vi "_Run Engine Server.vi"() -> ()   [LabVIEW 2015]
uses:
  Type/_Run State.ctl
  Type/_Log Command.ctl
  Type/_File Command.ctl
  Type/_RT Command.ctl
  Configuration/AcquisitionState.ctl
  _Server Global.vi
  Configuration/_Global Configuration.vi
panel:
  out "appended array":i32[](array[numeric])
  out "size(s)":i32
  out "first subarray":i32[](array[numeric])
  out "Remaining Scans":i32
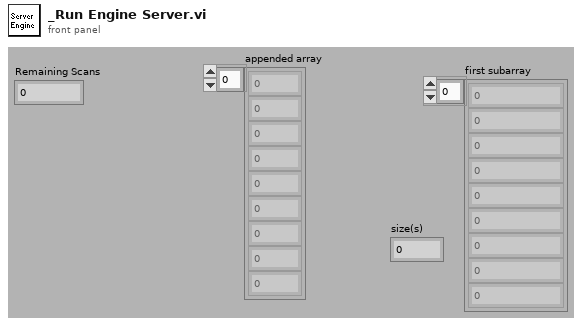
[diagram p1: front panel]
types:
  T1 = typedef "_Run State.ctl" = enum16{"Init", "Update", "Start", "End", "Error"}
  T2 = typedef "_Log Command.ctl" = enum16{"No Command", "Open", "Read", "Write", "Close", "Check Size"}
  T3 = typedef "_File Command.ctl" = enum16{"No Command", "Open", "Open Read", "Write", "Get Spectrum", "Close"}
  T4 = typedef "_RT Command.ctl" = enum16{"xml Start Run", "xml Start Actual Run", "xml Stop Run", "xml Runtime Update", "xml Get Status", "xml Get Table", "xml Set Table", "xml Get Configuration", "xml System Status", "xml Set LC Input Logic", "xml Get Data", "xml Get Info", "Start", "StartActualRun", "Stop", "Runtime Update", "Get Data", "Get Info", "Get Status", "Get Param", "Get Config", "Get Table", "Read ADC", "Set Oscillator", "Update Config", "Update Table", "Set All Pol", "Set Pol and DC", "Set Max Mass", "Toggle RP", "Toggle EL", "Set PIC", "Initialize Turbo", "Send Turbo Comm", "Close Turbo", "P1", "P2", "P3", "Send Serial", "Set LC Out", "Get LC In", "Read VAC", "Test Table", "Toggle Power", "Get Startup", "Set Startup", "Get ADC Table", "Set ADC Table", "Get Brief Status", "Get Detail Status", "Auxiliary Update", "Set CC Logics", "Set CC Input Logics", "Ignore Error", "invalid"}
  T5 = typedef "AcquisitionState.ctl" = enum16{"Ready", "Busy", "Waiting"}
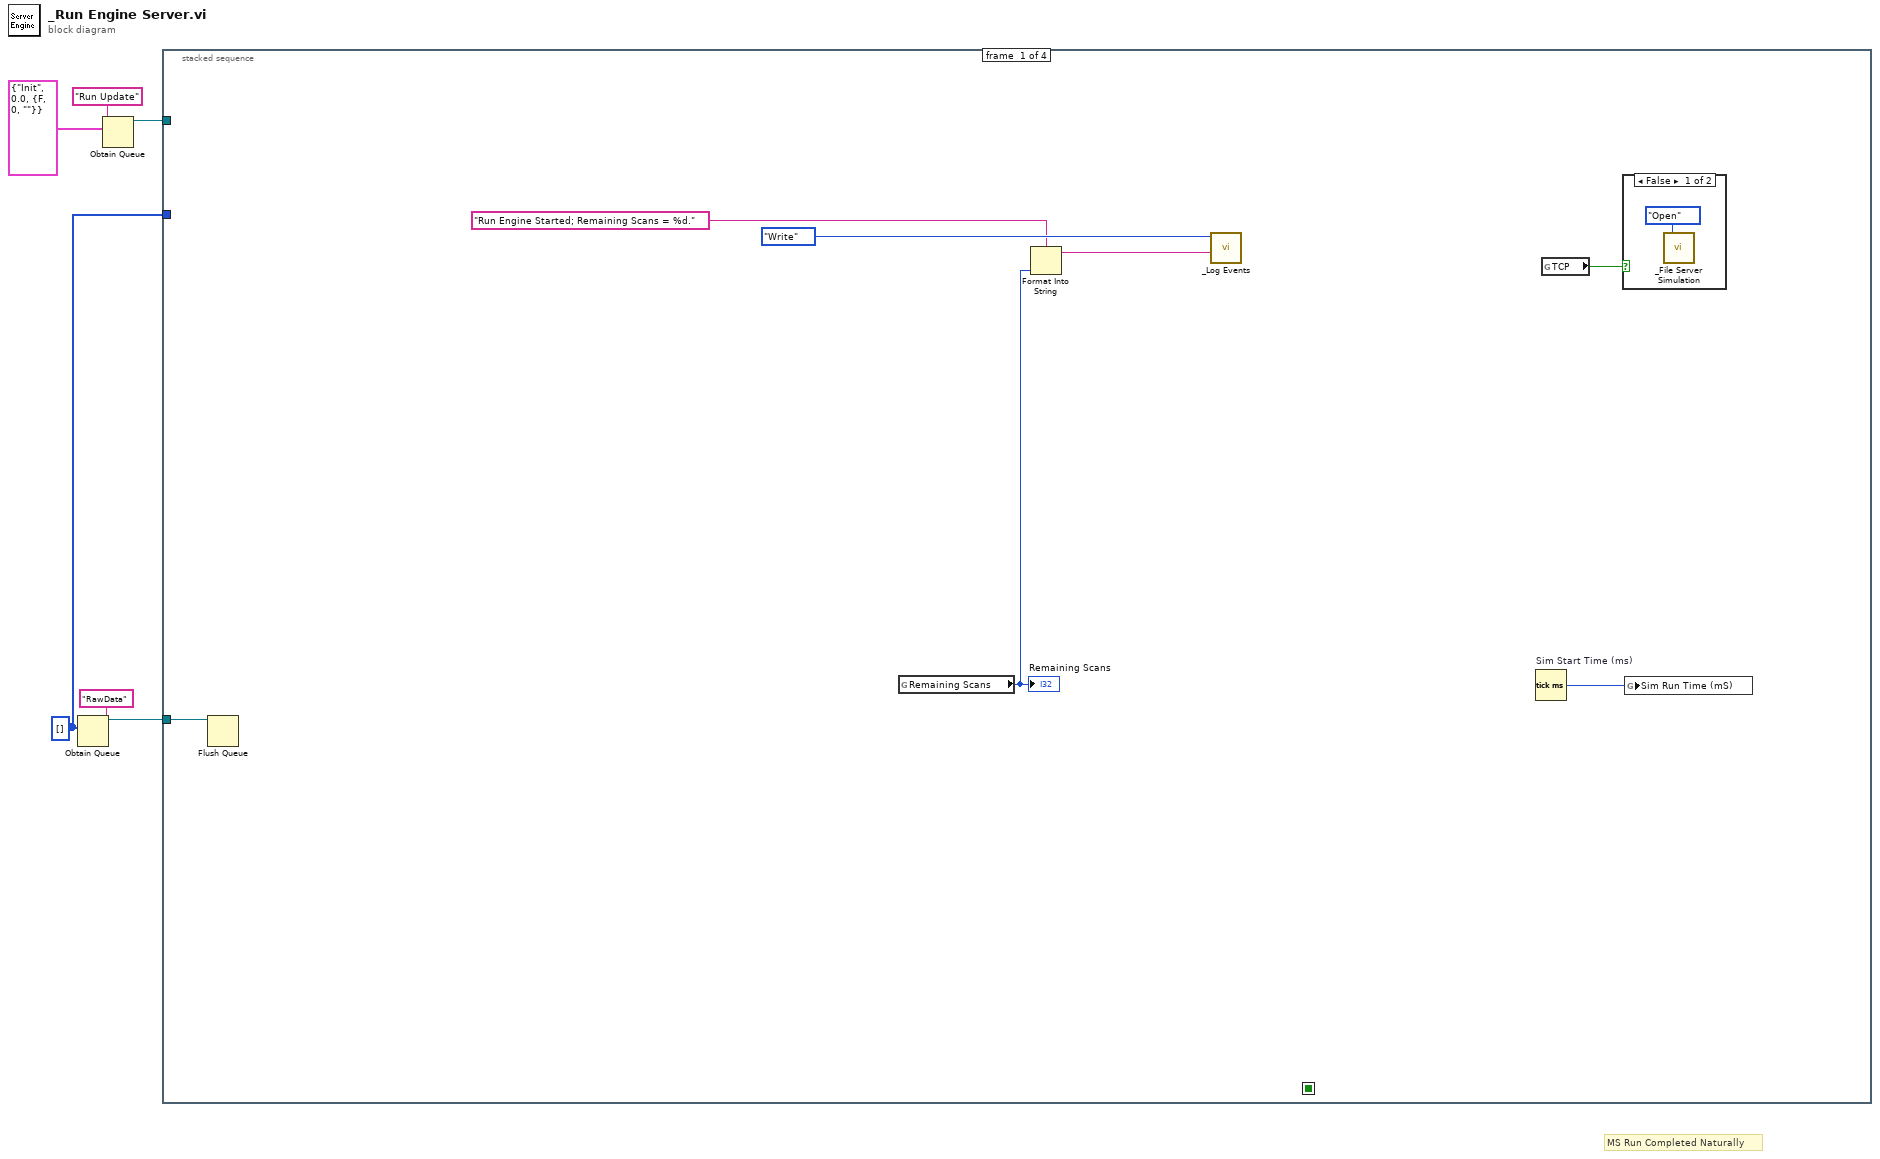
[diagram p0: block diagram]
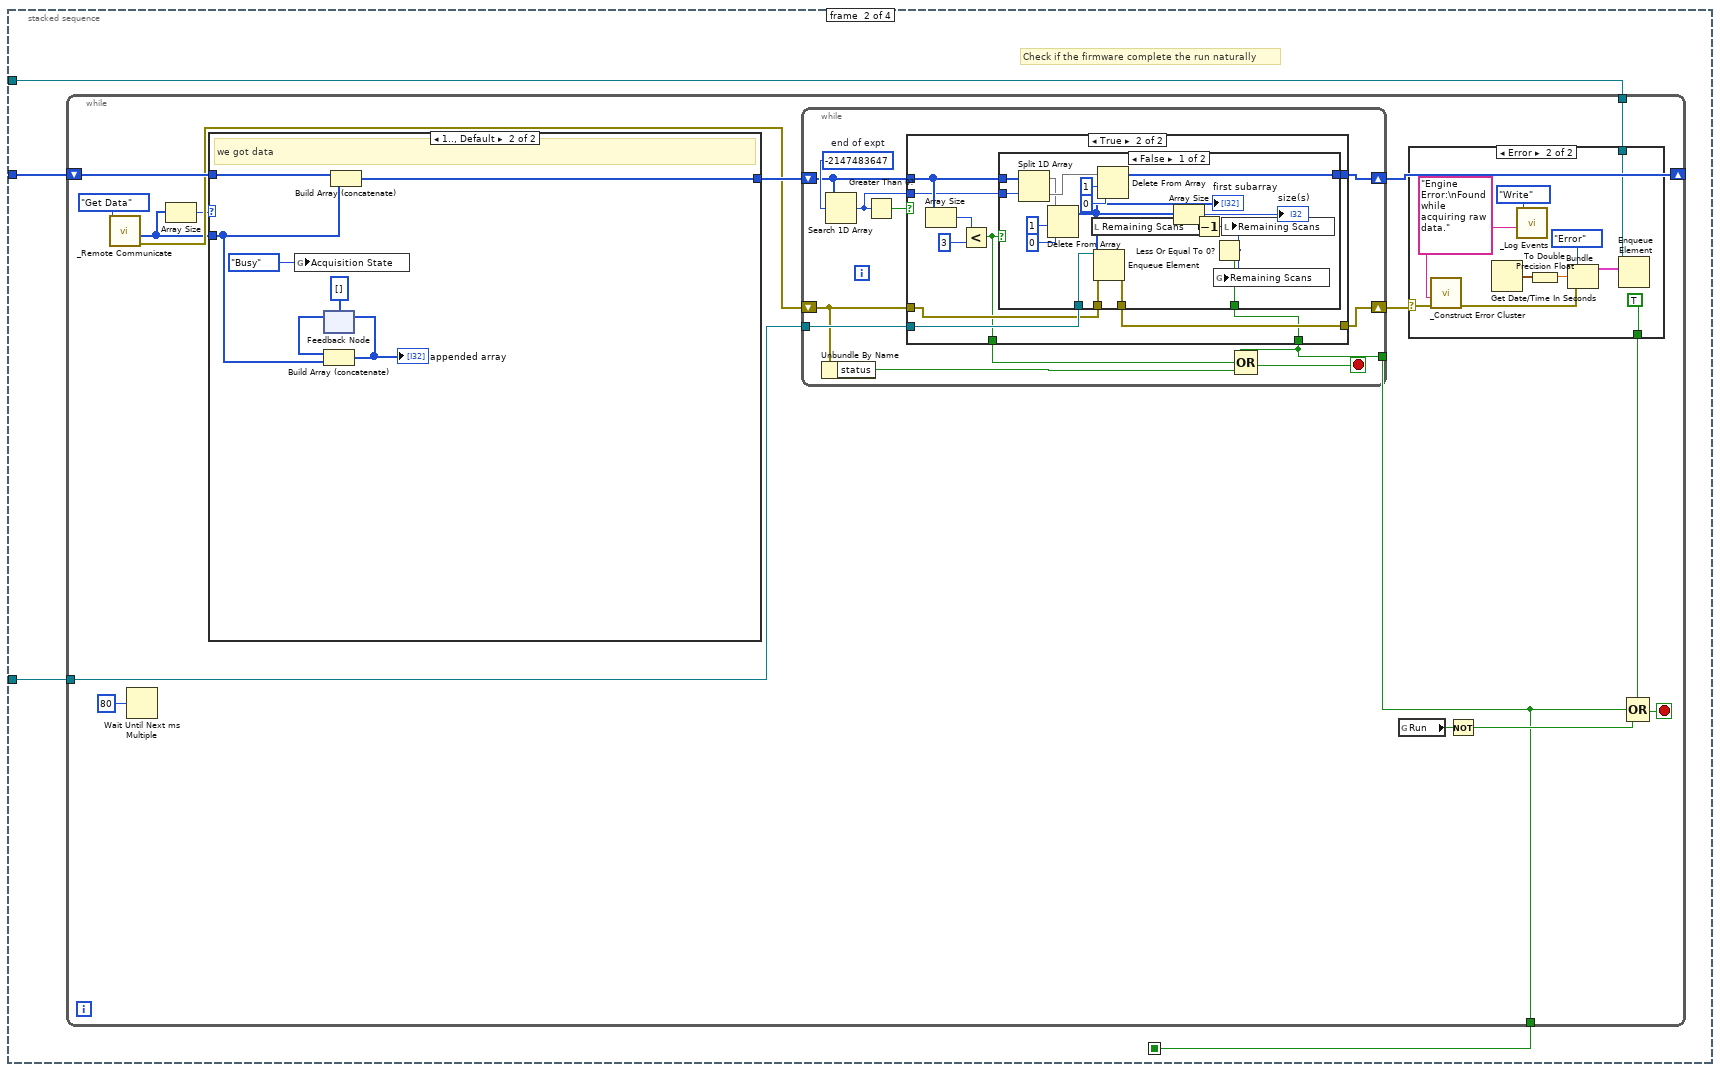
[diagram p3: hidden frame]
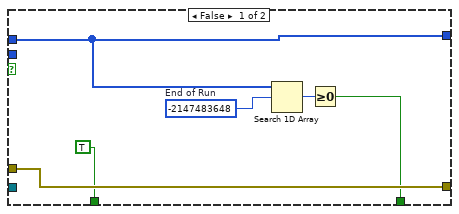
[diagram p5: hidden frame]
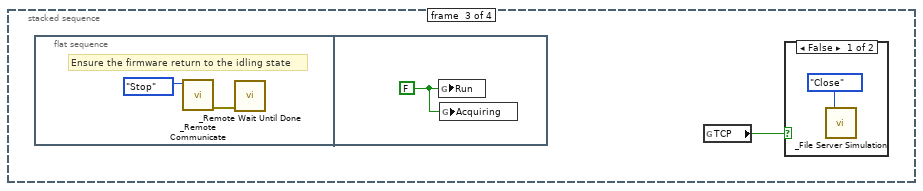
[diagram p8: hidden frame]
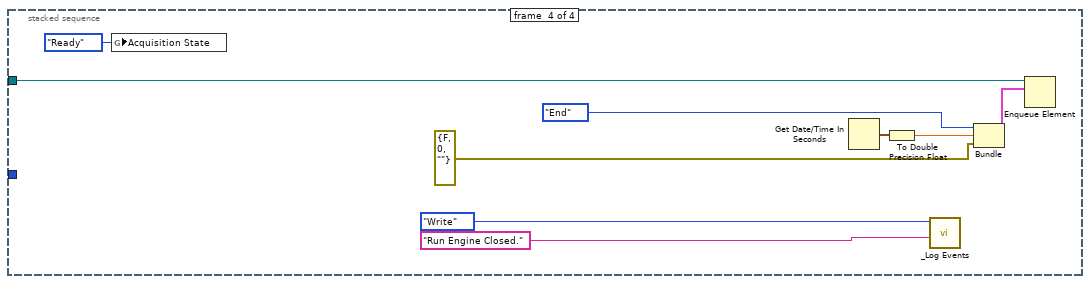
[diagram p10: hidden frame]
diagram:
  w4 = i32[] []
  # "MS Run Completed Naturally"
  n1 = Obtain Queue(name (unnamed)="RawData", element data type=w4) -> (queue out=w5:refnum<queue>)  [unwired: 3 in, 2 out]
  n2 = Obtain Queue(name (unnamed)="Run Update", element data type=cluster{T1, dbl, "error out":errorcluster} {enum."Init", 0.0, "error out"={"status"=FALSE, "code"=0, "source"=""}}) -> (queue out=w1:refnum<queue>)  [unwired: 3 in, 2 out]
  n3 = stacked-sequence {
    seq-local: [_ w15 _ _] -> [_ _ _ _]
    tunnel: w5 -> [w13 w18 _ _]
    tunnel: w4 -> [_ w17 _ _]
    tunnel: w1 -> [_ w16 _ w108]
    frame #0 {
      n4 = Flush Queue(queue=w13) -> ()  [unwired: 1 in, 3 out]
      n5 = global read "_Server Global.vi" "Remaining Scans"() -> (w11:i32)
      "Remaining Scans" <- w11
      n6 = Format Into String(format string="Run Engine Started; Remaining Scans = %d.", w11) -> (resulting string=w9:string)  [unwired: 2 in, 1 out]
      n7 = call "_Log Events.vi"("Event"=w9, "Log Command"=_Log_Command."Write") -> ()  [unwired: 6 in, 2 out]
      n8 = Tick Count (ms) "Sim Start Time (ms)"() -> (millisecond timer value=w7:u32)
      n9 = global read "_Global Configuration.vi" "TCP"() -> (w8:bool)
      n10 = case shown="False" w8 {
        frame False {
          n11 = call "_File Server Simulation.vi"("FileCommand"=_File_Command."Open") -> ()  [unwired: 1 in, 2 out]
        }
        frame True {
        }
      }
      n12 = global write "_Server Global.vi" "Sim Run Time (mS)"(w7) -> ()
    }
    frame #1 {
      # "Check if the firmware complete the run naturally"
      n13 = while {
        tunnel: w18 -> [w33]
        shift-right: [w27] -> _
        shift-left: w17 -> [w26]
        tunnel: w16 -> [w22]
        tunnel: [w21] -> w15
        stop <- w32 stop-if-true
        n14 = call "_Remote Communicate.vi"("Command"=_RT_Command."Get Data") -> ("error out"=w24:errorcluster, "Data Array"=w20:i32[])  [unwired: 5 in, 2 out]
        n15 = Wait Until Next ms Multiple(millisecond multiple=u32 80) -> ()  [unwired: 1 out]
        n16 = Array Size(array=w20) -> (size(s)=w19:i32)
        n17 = case shown="1.., Default" w19 {
          tunnel: w26 -> [w35 w42]
          tunnel: [w35 w41] -> w25
          tunnel: w20 -> [_ w36]
          frame 0 {
            # "nothing yet"
          }
          frame 1.., Default {
            # "we got data"
            n18 = global write "_Global Configuration.vi" "Acquisition State"(AcquisitionState."Busy" ("Acquisition State")) -> ()
            n19 = feedback #1(i32[] []) -> (w39:i32[])
            n20 = Build Array (concatenate)(w39, w36) -> (w38:i32[])
            "appended array" <- w38
            n21 = feedback-in #1(w38) -> ()
            n22 = Build Array (concatenate)(w42, w36) -> (w41:i32[])
          }
        }
        n23 = while {
          tunnel: w33 -> [w54]
          tunnel: [w46] -> w21
          shift-right: [w52] -> w27
          shift-left: w25 -> [w50]
          shift-right: [w53] -> w29
          shift-left: w24 -> [w48]
          stop <- w44 stop-if-true
          w51 = -2147483647  # end of expt
          n24 = Unbundle By Name(w48) -> ("status"=w45:bool)
          n25 = Search 1D Array(1D array=w50, element=w51) -> (index of element=w49:i32)  [unwired: 1 out]
          n26 = Greater Than 0?(x=w49) -> (x > 0?=w47:bool)
          n27 = case shown="True" w47 {
            tunnel: w48 -> [w60 w68]
            tunnel: w54 -> [_ w69]
            tunnel: [w60 w67] -> w53
            tunnel: w50 -> [w57 w63]
            tunnel: [w57 w70] -> w52
            tunnel: [w56 w66] -> w46
            tunnel: w49 -> [_ w62]
            tunnel: [TRUE w61] -> w43
            frame False {
              w58 = -2147483648  # End of Run
              n28 = Search 1D Array(1D array=w57, element=w58) -> (index of element=w59:i32)  [unwired: 1 out]
              n29 = Greater Or Equal To 0?(x=w59) -> (x >= 0?=w56:bool)
            }
            frame True {
              n30 = Array Size(array=w63) -> (size(s)=w65:i32)
              n31 = Less?(x=w65, y=3) -> (x < y?=w61:bool)
              n32 = case shown="False" w61 {
                tunnel: w63 -> [w87 w88]
                tunnel: w62 -> [w86 _]
                tunnel: [w79 w88] -> w70
                tunnel: w69 -> [w82 _]
                tunnel: w68 -> [w81 w89]
                tunnel: [w80 w89] -> w67
                tunnel: [w72 _] -> w66
                frame False {
                  n33 = Split 1D Array(array=w87, index=w86) -> (first subarray=w74:i32[], second subarray=w84:i32[])
                  n34 = Delete From Array(array=w74, length=1, index=0) -> (array with subset deleted=w73:i32[])  [unwired: 1 out]
                  "first subarray" <- w73
                  n35 = local read "Remaining Scans"() -> (w78:i32)
                  n36 = Enqueue Element(queue=w82, element=w73, error in (no error)=w81) -> (error out=w80:errorcluster)  [unwired: 3 out]
                  n37 = Delete From Array(array=w84, length=1, index=0) -> (array with subset deleted=w79:i32[])  [unwired: 1 out]
                  n38 = Array Size(array=w73) -> (size(s)=→"size(s)":i32)
                  n39 = Decrement(x=w78) -> (x-1=w71:i32)
                  n40 = Less Or Equal To 0?(x=w71) -> (x <= 0?=w72:bool)
                  n41 = global write "_Server Global.vi" "Remaining Scans"(w71) -> ()
                  n42 = local write "Remaining Scans"(w71) -> ()
                }
                frame True {
                }
              }
            }
          }
          n43 = Compound Arithmetic op=OR(w46, w43, w45) -> (w44:bool)
        }
        n44 = global read "_Global Configuration.vi" "Run"() -> (w31:bool)
        n45 = case shown="Error" w29 {
          selector: w29 -> [_ w99]
          tunnel: [_ TRUE] -> w28
          tunnel: w22 -> [_ w92]
          frame No Error {
          }
          frame Error {
            w90 = "Engine Error:\nFound while  acquiring raw data." ("format string")
            n46 = call "_Construct Error Cluster.vi"("error in"=w99, "reason"=w90) -> ("error out"=w95:errorcluster)  [unwired: 2 in, 3 out]
            n47 = Get Date/Time In Seconds() -> (seconds since 1Jan1904=w94:timestamp)
            n48 = call "_Log Events.vi"("Event"=w90, "Log Command"=_Log_Command."Write" ("File Command")) -> ()  [unwired: 6 in, 2 out]
            n49 = To Double Precision Float(number=w94) -> (double precision float=w93:dbl)
            n50 = Bundle(_Run_State."Error", w93, "error out"=w95) -> (w97:cluster{T1, dbl, "error out":errorcluster})  [unwired: 1 out]
            n51 = Enqueue Element(queue=w92, element=w97) -> ()  [unwired: 1 in, 4 out]
          }
        }
        n52 = Not(x=w31) -> (.not. x?=w30:bool)
        n53 = Compound Arithmetic op=OR(w28, w21, w30) -> (w32:bool)
      }
    }
    frame #2 {
      n54 = flat-sequence {
        frame #0 {
          # "Ensure the firmware return to the idling state"
          n55 = call "_Remote Communicate.vi"("Command"=_RT_Command."Stop") -> ("error out"=w103:errorcluster)  [unwired: 5 in, 3 out]
          n56 = call "_Remote Wait Until Done.vi"("error IO"=w103) -> ()  [unwired: 1 in, 2 out]
        }
        frame #1 {
          w104 = FALSE ("Update")
          n57 = global write "_Global Configuration.vi" "Run"(w104) -> ()
          n58 = global write "_Global Configuration.vi" "Acquiring"(w104) -> ()
        }
      }
      n59 = global read "_Global Configuration.vi" "TCP"() -> (w100:bool)
      n60 = case shown="False" w100 {
        frame False {
          n61 = call "_File Server Simulation.vi"("FileCommand"=_File_Command."Close") -> ()  [unwired: 1 in, 2 out]
        }
        frame True {
        }
      }
    }
    frame #3 {
      n62 = global write "_Global Configuration.vi" "Acquisition State"(AcquisitionState."Ready" ("Acquisition State")) -> ()
      n63 = Get Date/Time In Seconds() -> (seconds since 1Jan1904=w109:timestamp)
      n64 = To Double Precision Float(number=w109) -> (double precision float=w111:dbl)
      n65 = call "_Log Events.vi"("Event"="Run Engine Closed." ("name (unnamed)"), "Log Command"=_Log_Command."Write") -> ()  [unwired: 6 in, 2 out]
      n66 = Bundle(_Run_State."End", w111, "error out"=errorcluster {"status"=FALSE, "code"=0, "source"=""}) -> (w110:cluster{T1, dbl, "error out":errorcluster})  [unwired: 1 out]
      n67 = Enqueue Element(queue=w108, element=w110) -> ()  [unwired: 1 in, 4 out]
    }
  }
